vi "Kstar单相电界面.vi"() -> ()   [LabVIEW 2016, in "环境动力监测库.lvlib" / "UPS库.lvlib"]
panel:
  out "x+1":u32
  in  "解除告警":bool
  out "状态":T1
  out "通信":bool=TRUE
  out "串口":string
  in  "查看型号":bool
  out "关机倒计时":i32
  out "关闭中":bool
  out "UPS状态":T2
  in  "关机":bool
  in  "重开串口":bool
  # "输入电压"
  # "V"
  # "V"
  # "输入故障电压"
  # "输出电压"
  # "V"
  # "输出电流"
  # "A"
  # "输入频率"
  # "Hz"
  # "电池电压"
  # "V"
  # "UPS温度"
  # "℃"
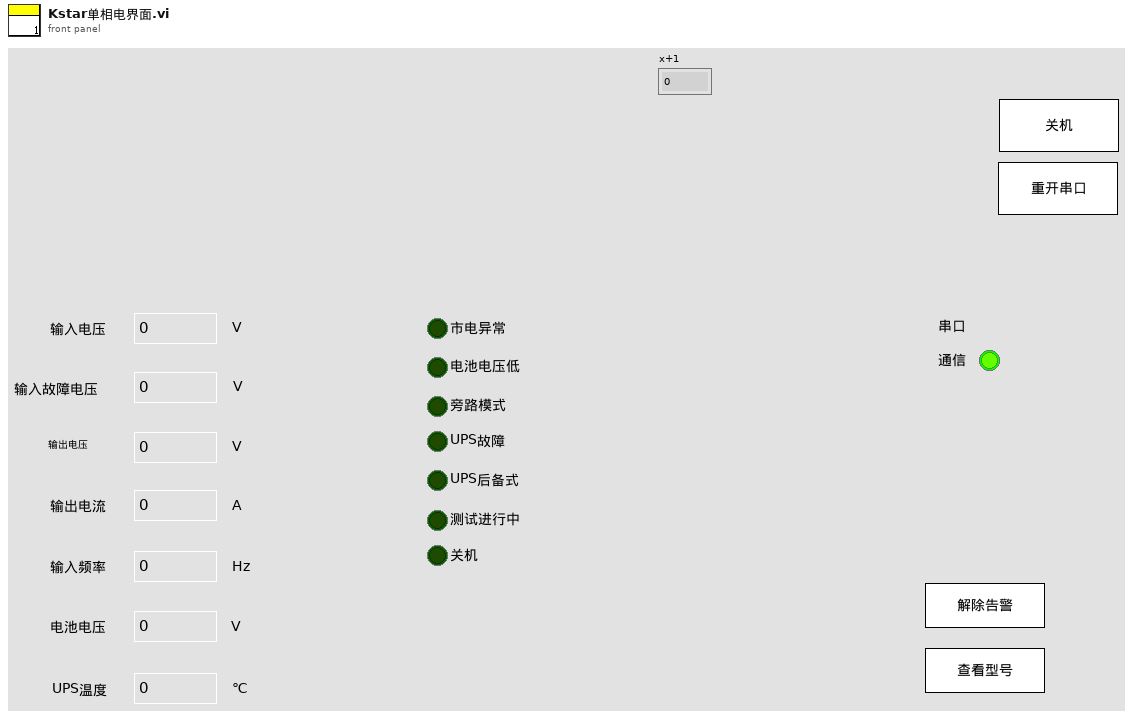
[diagram p1: front panel]
types:
  T1 = cluster{"I/P voltage":dbl, "I/P fault voltage":dbl, "O/P voltage":dbl, "O/P load %":dbl, "I/P frequency HZ":dbl, "Battery voltage":dbl, "Temperature":dbl}
  T2 = cluster{"市电异常":bool, "电池电压低":bool, "旁路模式":bool, "UPS故障":bool, "UPS后备式":bool, "测试进行中":bool, "关机":bool, "保留":bool}
  T3 = cluster{"枚举":enum16{"open", "read", "write", "close"}, "写入缓冲区":string}
  T4 = enum32{"Bad", "Idle", "Run top level", "Running"}
  T5 = cluster{"漏水监测输出":cluster{"漏水监测告警":bool, "告警内容":string}, "门禁监测输出":cluster{"门禁监测告警":bool, "告警内容":string}, "门禁监测输出2":cluster{"门禁监测告警":bool, "告警内容":string}, "温湿度监测输出":cluster{"温湿度监测告警":bool, "告警内容":string}, "烟雾监测输出":cluster{"烟雾监测告警":bool, "告警内容":string}, "空调监测输出":cluster{"空调监测告警":bool, "告警内容":string}, "自动重合闸输出":cluster{"自动重合闸告警":bool, "告警内容":string}, "红外入侵输出":cluster{"红外入侵告警":bool, "告警内容":string}, "振动输出":cluster{"振动告警":bool, "告警内容":string}, "UPS输出":cluster{"UPS告警":bool, "告警内容":string}, "蓄电池输出":cluster{"蓄电池告警":bool, "告警内容":string}, "蓄电池输出2":cluster{"蓄电池告警":bool, "告警内容":string}, "GPS输出":cluster{"定位告警":bool, "告警内容":string}, "北斗输出":cluster{"定位告警":bool, "告警内容":string}, "气象输出":cluster{"气象告警":bool, "告警内容":string}, "废液输出":cluster{"废液告警":bool, "告警内容":string}, "废液输出2":cluster{"废液告警":bool, "告警内容":string}, "灭火装置输出":cluster{"灭火装置告警":bool, "告警内容":string}}
  T6 = typedef "环境动力监测库.lvlib/UPS库.lvlib/UPS型号.ctl" = enum16{"山特UPSC1~3", "山特UPSC6~20", "华为UPS2000-G-(1-3KVA)", "Kstar"}
  T7 = cluster{"VISA resource name":refnum<visa-resource-name>, "Serial Config":cluster{"baud rate (9600)":u32, "stop bits (10: 1 bit)":u16, "parity (0:none)":enum16{"None", "Odd", "Even", "Mark", "Space"}, "data bits (8)":u16, "timeout (10sec)":u32}, "型号选择":T6, "HW-UPS-2000 MB session":refnum<class "MB_Master.lvclass">, "连接方式":enum16{"串口", "TCP"}, "IP":string, "Port":string, "低电量报警阈值":u16, "功能启用":bool}
  T8 = cluster{"I/P voltage":dbl, "I/P fault voltage":dbl, "O/P voltage":dbl, "O/P load %":dbl, "I/P frequency HZ":dbl, "Battery voltage":dbl, "Temperature":dbl, "U":string}
  T9 = cluster{"市电":cluster{"状态":bool, "电压:":u16, "电流：":dbl, "详情  ":bool}, "UPS":cluster{"状态":bool, "输入电压:":sgl, "输出电压:":sgl, "电池电量:":u8, "电量":u16, "详情  ":bool}, "蓄电池12V":cluster{"状态":bool, "电压:":sgl, "电流:":sgl, "电池电量:":u8, "电量":u16, "详情  ":bool, "充电":bool, "负载":bool}, "蓄电池24V":cluster{"状态":bool, "电压:":sgl, "电流:":sgl, "电池电量:":u8, "电量":u16, "详情  ":bool, "充电":bool, "负载":bool}}
  T10 = cluster{"[0]":bool, "[1]":bool, "[2]":bool, "[3]":bool, "[4]":bool, "[5]":bool, "[6]":bool, "[7]":bool}
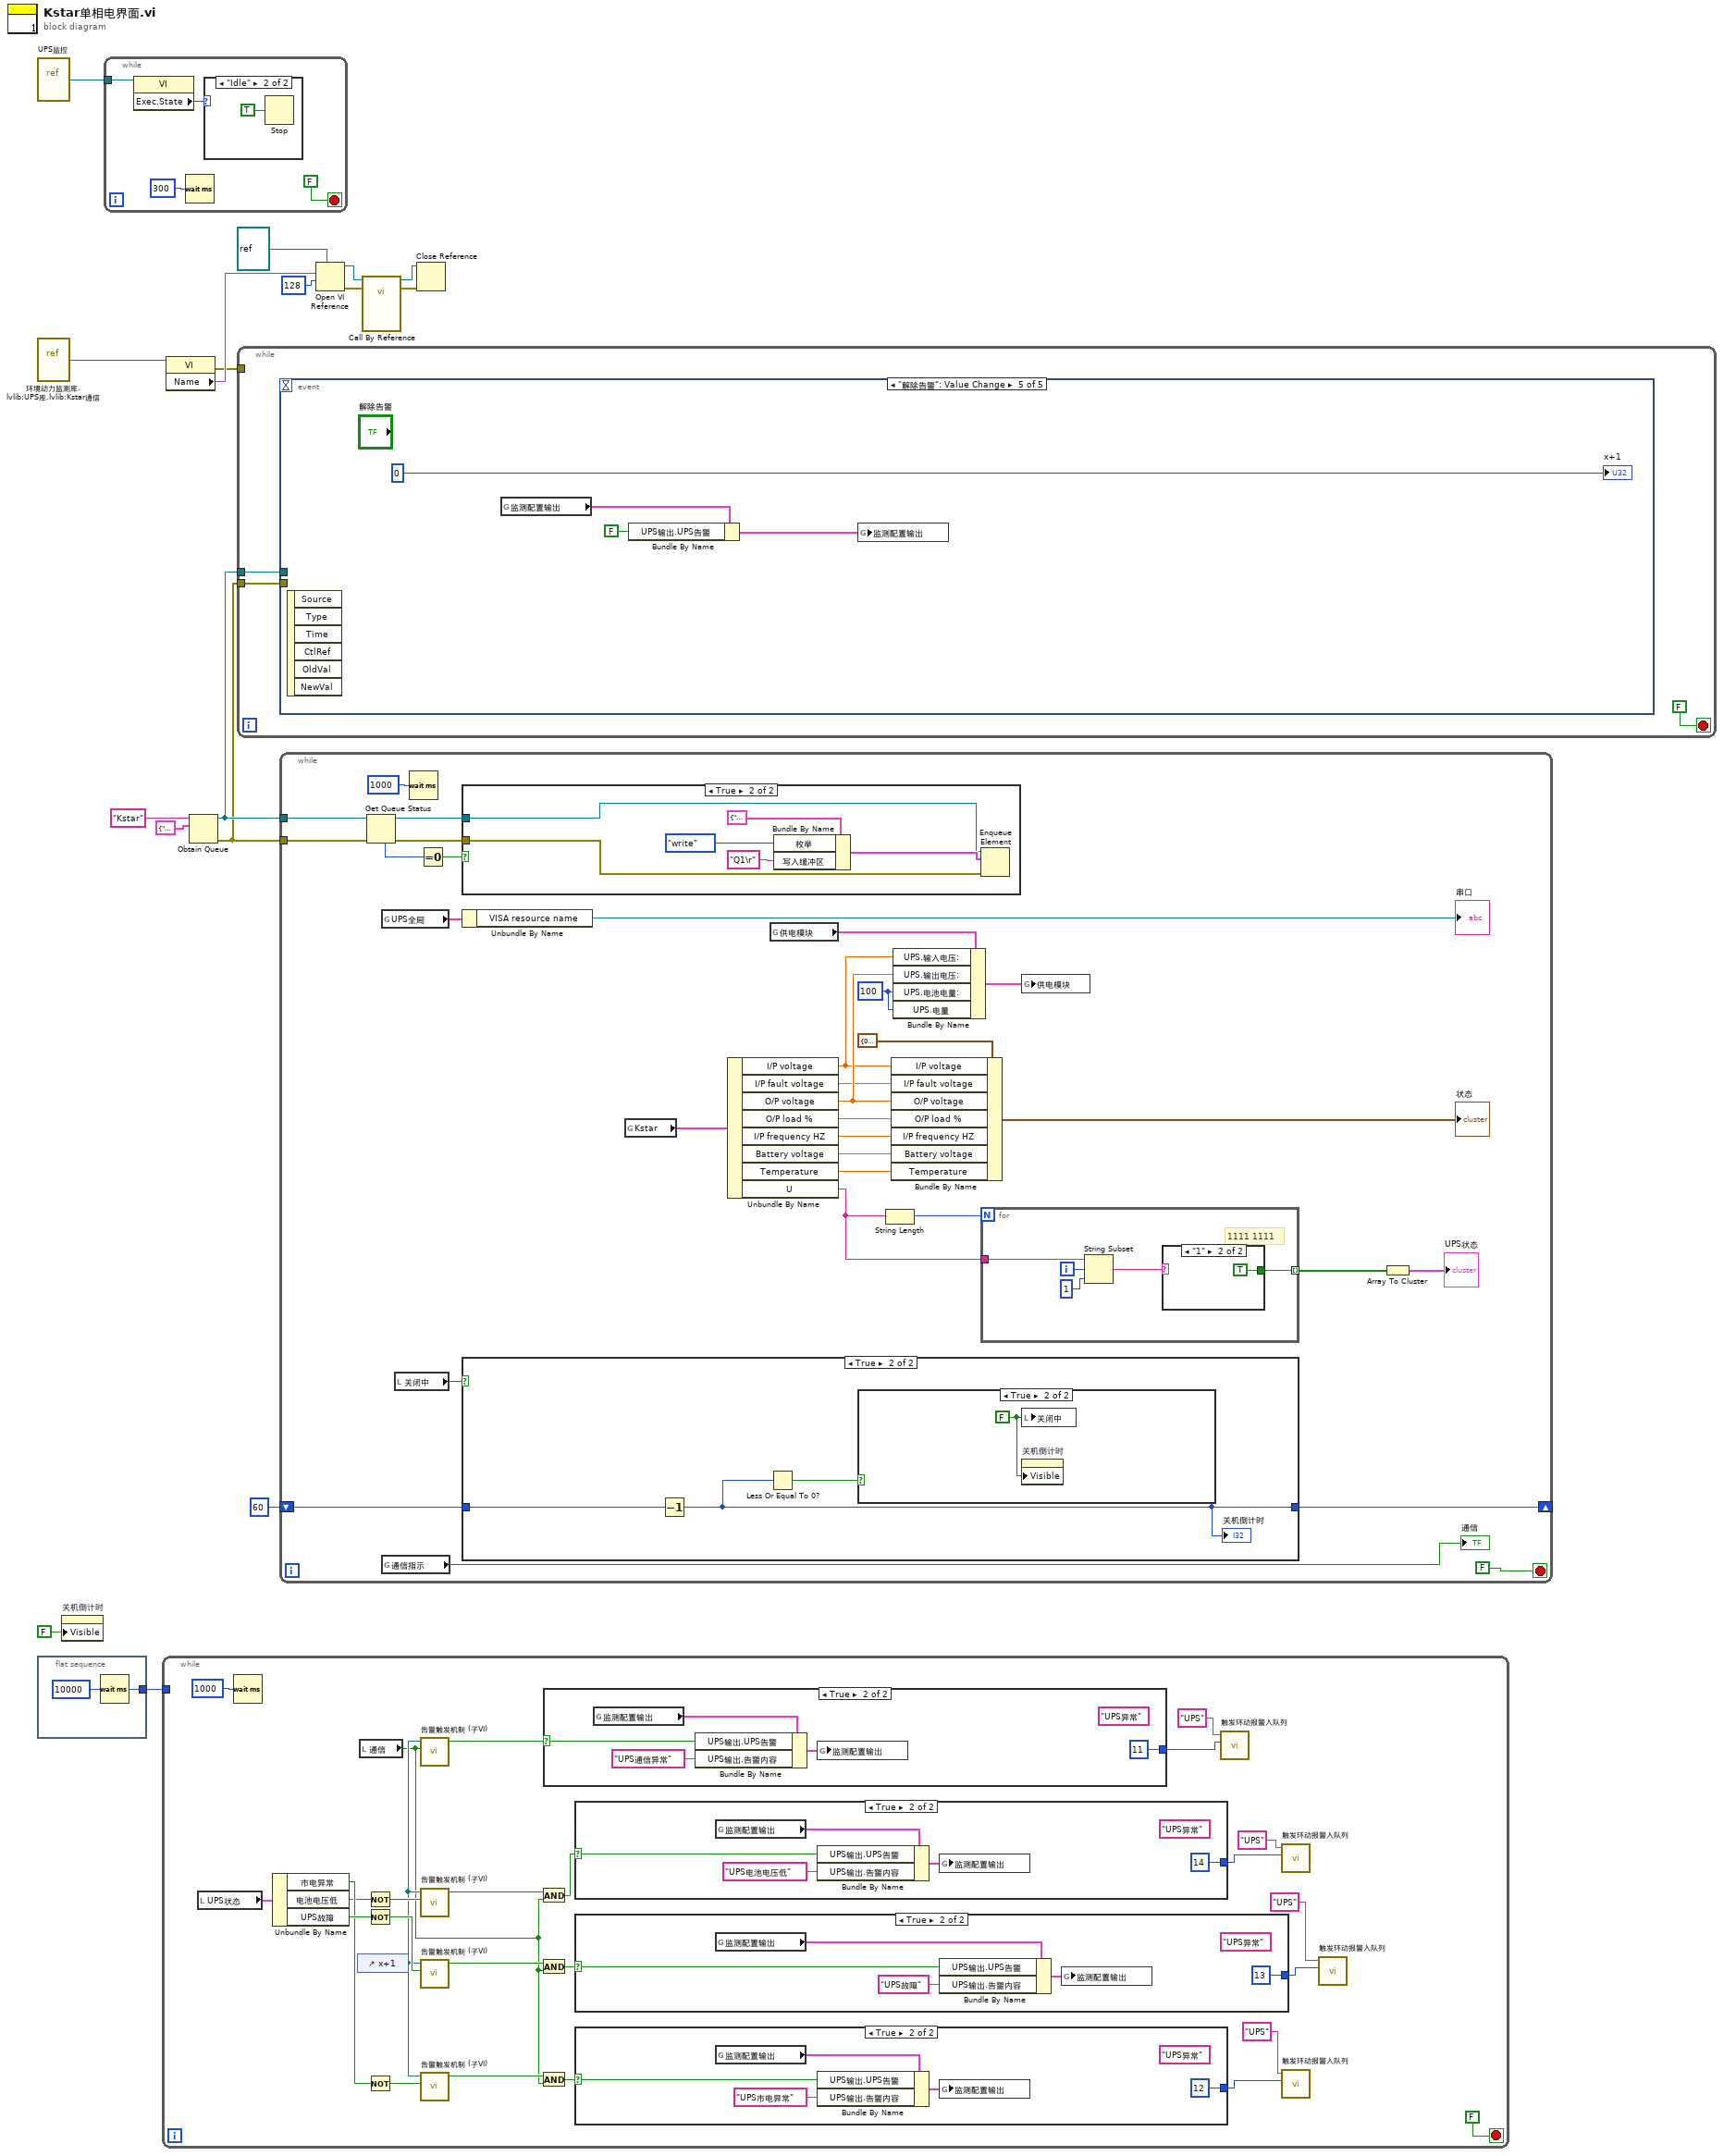
[diagram p0: block diagram]
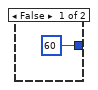
[diagram p8: hidden frame]
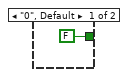
[diagram p10: hidden frame]
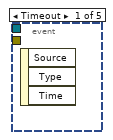
[diagram p11: hidden frame]
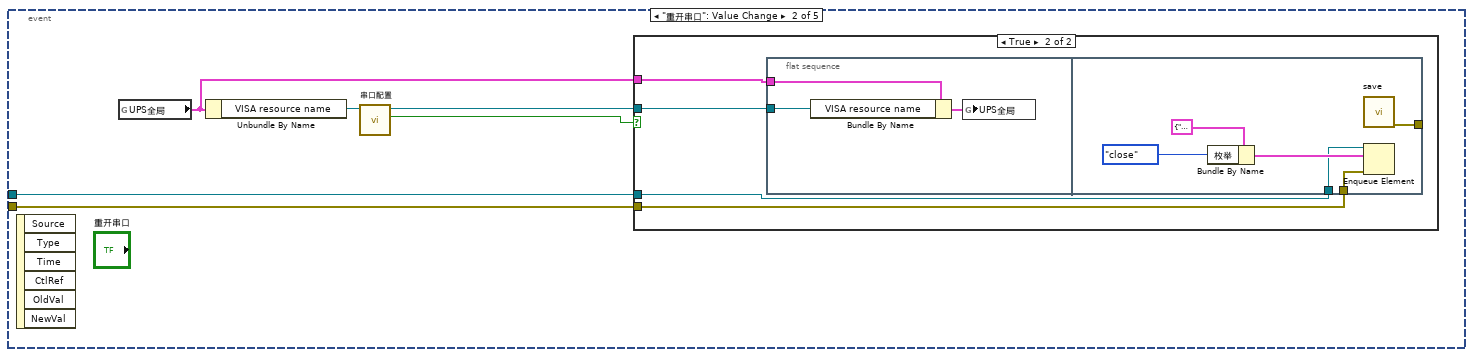
[diagram p12: hidden frame]
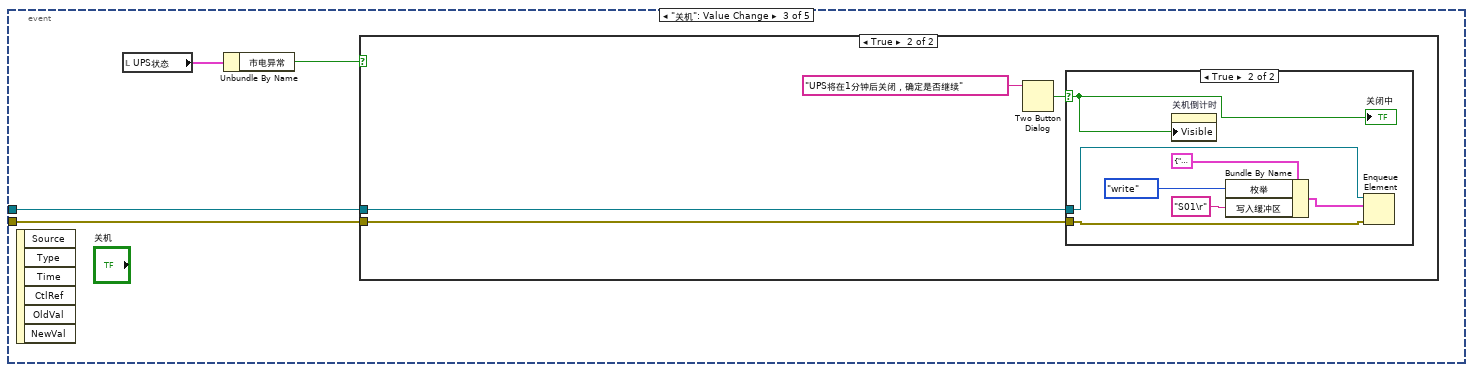
[diagram p14: hidden frame]
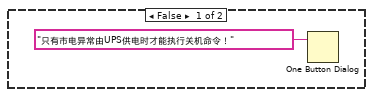
[diagram p15: hidden frame]
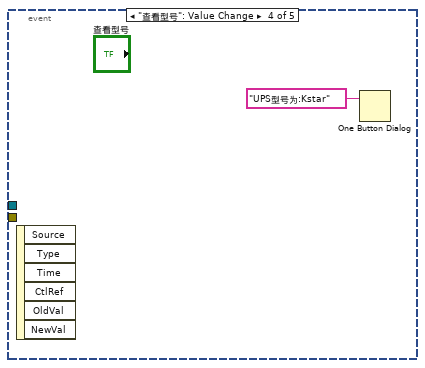
[diagram p17: hidden frame]
diagram:
  n1 = vi-ref "UPS监控.vi"() -> (w2:refnum<vi>)
  n2 = vi-ref "环境动力监测库.lvlib:UPS库.lvlib:Kstar通信.vi"() -> (w10:refnum<vi>)
  n3 = flat-sequence {
    tunnel: [w18] -> w1
    frame #0 {
      n4 = Wait (ms)(milliseconds to wait=u32 10000 ("等待时间（毫秒）")) -> (millisecond timer value=w18:u32)
    }
  }
  n5 = property on="关机倒计时" class="DigNum (strict)"("Visible"=FALSE ("可见")) -> ()  [unwired: 2 in, 2 out]
  n6 = while {
    tunnel: w2 -> [w23]
    stop <- FALSE stop-if-true
    n7 = property class="VI"(reference=w23) -> ("Exec.State"=w22:T4)  [unwired: 1 in, 2 out]
    n8 = Wait (ms)(milliseconds to wait=u32 300 ("等待时间（毫秒）")) -> ()  [unwired: 1 out]
    n9 = case shown="\"Idle\"" w22 {
      frame "Bad", Default {
      }
      frame "Idle" {
        n10 = Stop(stop? (T)=TRUE ("停止？(T)")) -> ()
      }
    }
  }
  n11 = while {
    tunnel: w1 -> [_]
    stop <- FALSE stop-if-true
    n12 = local read "UPS状态"() -> (w48:T2)
    n13 = Wait (ms)(milliseconds to wait=u32 1000 ("等待时间（毫秒）")) -> ()  [unwired: 1 out]
    n14 = Unbundle By Name(w48) -> ("市电异常"=w42:bool, "电池电压低"=w39:bool, "UPS故障"=w45:bool)
    n15 = control-ref of="x+1"() -> (w37:refnum<vi>)
    n16 = local read "通信"() -> (w33:bool)
    n17 = Not(x=w39) -> (.not. x?=w40:bool)
    n18 = Not(x=w45) -> (.not. x?=w46:bool)
    n19 = Not(x=w42) -> (.not. x?=w43:bool)
    n20 = call "告警触发机制 (子VI).vi"("状态输出真-正常"=w33, "Digital输入"=w37) -> ("触发告警"=w47:bool)  [unwired: 7 in, 2 out]
    n21 = call "告警触发机制 (子VI).vi"("状态输出真-正常"=w40, "Digital输入"=w37) -> ("触发告警"=w38:bool)  [unwired: 7 in, 2 out]
    n22 = call "告警触发机制 (子VI).vi"("状态输出真-正常"=w46, "Digital输入"=w37) -> ("触发告警"=w44:bool)  [unwired: 7 in, 2 out]
    n23 = call "告警触发机制 (子VI).vi"("状态输出真-正常"=w43, "Digital输入"=w37) -> ("触发告警"=w41:bool)  [unwired: 7 in, 2 out]
    n24 = And(x=w38, y=w33) -> (x .and. y?=w35:bool)
    n25 = And(x=w44, y=w33) -> (x .and. y?=w34:bool)
    n26 = And(x=w41, y=w33) -> (x .and. y?=w36:bool)
    n27 = case shown="True" w47 {
      selector: w47 -> [_ w55]
      tunnel: [_ 11 ("code")] -> w32
      frame False {
      }
      frame True {
        (unwired) "UPS异常" ("设备")
        n28 = global read "内部交互全局变量.vi" "监测配置输出"() -> (w53:T5)
        n29 = Bundle By Name(cluster=w53, "UPS输出.UPS告警"=w55, "UPS输出.告警内容"="UPS通信异常" ("报警内容")) -> (w54:T5)
        n30 = global write "内部交互全局变量.vi" "监测配置输出"(w54) -> ()
      }
    }
    n31 = case shown="True" w35 {
      selector: w35 -> [_ w65]
      tunnel: [_ 14 ("code")] -> w29
      frame False {
      }
      frame True {
        (unwired) "UPS异常" ("设备")
        n32 = global read "内部交互全局变量.vi" "监测配置输出"() -> (w64:T5)
        n33 = Bundle By Name(cluster=w64, "UPS输出.UPS告警"=w65, "UPS输出.告警内容"="UPS电池电压低" ("报警内容")) -> (w63:T5)
        n34 = global write "内部交互全局变量.vi" "监测配置输出"(w63) -> ()
      }
    }
    n35 = case shown="True" w34 {
      selector: w34 -> [_ w60]
      tunnel: [_ 13 ("code")] -> w28
      frame False {
      }
      frame True {
        (unwired) "UPS异常" ("设备")
        n36 = global read "内部交互全局变量.vi" "监测配置输出"() -> (w59:T5)
        n37 = Bundle By Name(cluster=w59, "UPS输出.UPS告警"=w60, "UPS输出.告警内容"="UPS故障" ("报警内容")) -> (w58:T5)
        n38 = global write "内部交互全局变量.vi" "监测配置输出"(w58) -> ()
      }
    }
    n39 = case shown="True" w36 {
      selector: w36 -> [_ w70]
      tunnel: [_ 12 ("code")] -> w27
      frame False {
      }
      frame True {
        (unwired) "UPS异常" ("设备")
        n40 = global read "内部交互全局变量.vi" "监测配置输出"() -> (w69:T5)
        n41 = Bundle By Name(cluster=w69, "UPS输出.UPS告警"=w70, "UPS输出.告警内容"="UPS市电异常" ("报警内容")) -> (w68:T5)
        n42 = global write "内部交互全局变量.vi" "监测配置输出"(w68) -> ()
      }
    }
    n43 = call "触发环动报警入队列.vi"("code"=w32, "元器件"="UPS" ("设备")) -> ()  [unwired: 10 in]
    n44 = call "触发环动报警入队列.vi"("code"=w29, "元器件"="UPS" ("设备")) -> ()  [unwired: 10 in]
    n45 = call "触发环动报警入队列.vi"("code"=w27, "元器件"="UPS" ("设备")) -> ()  [unwired: 10 in]
    n46 = call "触发环动报警入队列.vi"("code"=w28, "元器件"="UPS" ("设备")) -> ()  [unwired: 10 in]
  }
  n47 = property class="VI"(reference=w10) -> (error out=w4:errorcluster, "Name"=w11:string)  [unwired: 1 in, 1 out]
  n48 = Obtain Queue(name (unnamed)="Kstar" ("名称（未命名）"), element data type=T3 {"枚举"=enum."open", "写入缓冲区"=""}) -> (queue out=w7:refnum<queue>, error out=w6:errorcluster)  [unwired: 3 in, 1 out]
  n49 = while {
    tunnel: w6 -> [w72]
    tunnel: w7 -> [w71]
    tunnel: w4 -> [_]
    stop <- FALSE stop-if-true
    n50 = event shown="[4] \"解除告警\": Value Change" {
      selector: _ -> [_ _ _ _ _]
      dyn-events: _ -> [_ _ _ _ _]
      timeout: _ -> [_ _ _ _ _]
      tunnel: w72 -> [_ w76 w95 _ _]
      tunnel: w71 -> [_ w77 w96 _ _]
      event Timeout {
        n51 = event-data() -> ()  [unwired: 1 in, 3 out]
      }
      event "重开串口": Value Change {
        n52 = event-data() -> ()  [unwired: 1 in, 6 out]
        n53 = global read "断电保存全局变量.vi" "UPS全局"() -> (w74:T7)
        n54 = Unbundle By Name(w74) -> ("VISA resource name"=w75:refnum<visa-resource-name>)
        n55 = call "串口配置.vi"("请选择串口:"=w75) -> ("确认 2"=w79:bool, "请选择串口: 2"=w78:refnum<visa-resource-name>)  [unwired: 9 in]
        n56 = case shown="True" w79 {
          tunnel: w78 -> [_ w83]
          tunnel: w77 -> [_ w82]
          tunnel: w76 -> [_ w81]
          tunnel: w74 -> [_ w80]
          frame False {
          }
          frame True {
            n57 = flat-sequence {
              tunnel: w83 -> [w84]
              tunnel: w80 -> [w86]
              tunnel: w82 -> [w89]
              tunnel: w81 -> [w88]
              tunnel: [w87] -> _
              frame #0 {
                n58 = Bundle By Name(cluster=w86, "VISA resource name"=w84) -> (w85:T7)
                n59 = global write "断电保存全局变量.vi" "UPS全局"(w85) -> ()
              }
              frame #1 {
                n60 = Bundle By Name(cluster=T3 {"枚举"=enum."open", "写入缓冲区"=""}, "枚举"=enum16{"open", "read", "write", "close"}."close") -> (w92:T3)
                n61 = call "save.vi"() -> ("error out"=w87:errorcluster)  [unwired: 11 in]
                n62 = Enqueue Element(queue=w89, element=w92, error in (no error)=w88) -> ()  [unwired: 1 in, 3 out]
              }
            }
          }
        }
      }
      event "关机": Value Change {
        n63 = event-data() -> ()  [unwired: 1 in, 6 out]
        n64 = local read "UPS状态"() -> (w94:T2)
        n65 = Unbundle By Name(w94) -> ("市电异常"=w93:bool)
        n66 = case shown="True" w93 {
          tunnel: w96 -> [_ w101]
          tunnel: w95 -> [_ w100]
          frame False {
            n67 = One Button Dialog(message="只有市电异常由UPS供电时才能执行关机命令！" ("消息")) -> ()  [unwired: 1 in, 1 out]
          }
          frame True {
            n68 = Two Button Dialog(message="UPS将在1分钟后关闭，确定是否继续" ("消息")) -> (T button?=w98:bool)  [unwired: 2 in]
            n69 = case shown="True" w98 {
              selector: w98 -> [_ w102]
              tunnel: w101 -> [_ w105]
              tunnel: w100 -> [_ w104]
              frame False {
              }
              frame True {
                n70 = property on="关机倒计时" class="DigNum (strict)"("Visible"=w102) -> ()  [unwired: 2 in, 2 out]
                n71 = Bundle By Name(cluster=T3 {"枚举"=enum."open", "写入缓冲区"=""}, "枚举"=enum16{"open", "read", "write", "close"}."write", "写入缓冲区"="S01\r") -> (w106:T3)
                n72 = Enqueue Element(queue=w105, element=w106, error in (no error)=w104) -> ()  [unwired: 1 in, 3 out]
                "关闭中" <- w102
              }
            }
          }
        }
      }
      event "查看型号": Value Change {
        n73 = event-data() -> ()  [unwired: 1 in, 6 out]
        n74 = One Button Dialog(message="UPS型号为:Kstar" ("消息")) -> ()  [unwired: 1 in, 1 out]
      }
      event "解除告警": Value Change {
        n75 = event-data() -> ()  [unwired: 1 in, 6 out]
        n76 = global read "内部交互全局变量.vi" "监测配置输出"() -> (w111:T5)
        n77 = Bundle By Name(cluster=w111, "UPS输出.UPS告警"=FALSE) -> (w110:T5)
        n78 = global write "内部交互全局变量.vi" "监测配置输出"(w110) -> ()
        "x+1" <- u32 0 ("x+1")
      }
    }
  }
  n79 = while {
    tunnel: w7 -> [w134]
    tunnel: w6 -> [w133]
    shift-right: [w136] -> _
    shift-left: 60 -> [w137]
    stop <- FALSE stop-if-true
    w127 = u8 100 ("UPS.电池电量:")
    n80 = Get Queue Status(queue=w134, error in (no error)=w133) -> (queue out=w132:refnum<queue>, error out=w131:errorcluster, # elements in queue=w135:i32)  [unwired: 1 in, 5 out]
    n81 = global read "断电保存全局变量.vi" "UPS全局"() -> (w115:T7)
    n82 = global read "UPS内部交互全局.vi" "通信指示"() -> (→"通信":bool)
    n83 = local read "关闭中"() -> (w138:bool)
    n84 = Wait (ms)(milliseconds to wait=u32 1000 ("等待时间（毫秒）")) -> ()  [unwired: 1 out]
    n85 = Equal To 0?(x=w135) -> (x = 0?=w130:bool)
    n86 = case shown="True" w130 {
      tunnel: w132 -> [_ w146]
      tunnel: w131 -> [_ w145]
      frame False {
      }
      frame True {
        n87 = Bundle By Name(cluster=T3 {"枚举"=enum."open", "写入缓冲区"=""}, "枚举"=enum16{"open", "read", "write", "close"}."write", "写入缓冲区"="Q1\r") -> (w149:T3)
        n88 = Enqueue Element(queue=w146, element=w149, error in (no error)=w145) -> ()  [unwired: 1 in, 3 out]
      }
    }
    n89 = Unbundle By Name(w115) -> ("VISA resource name"=→"串口":refnum<visa-resource-name>)
    n90 = case shown="True" w138 {
      tunnel: w137 -> [_ w154]
      tunnel: [60 w153] -> w136
      frame False {
      }
      frame True {
        n91 = Decrement(x=w154) -> (x-1=w153:i32)
        "关机倒计时" <- w153
        n92 = Less Or Equal To 0?(x=w153) -> (x <= 0?=w152:bool)
        n93 = case shown="True" w152 {
          frame False {
          }
          frame True {
            w155 = FALSE ("关闭中")
            n94 = local write "关闭中"(w155) -> ()
            n95 = property on="关机倒计时" class="DigNum (strict)"("Visible"=w155) -> ()  [unwired: 2 in, 2 out]
          }
        }
      }
    }
    n96 = global read "UPS内部交互全局.vi" "Kstar"() -> (w142:T8)
    n97 = Unbundle By Name(w142) -> ("I/P voltage"=w117:dbl, "I/P fault voltage"=w116:dbl, "O/P voltage"=w118:dbl, "O/P load %"=w119:dbl, "I/P frequency HZ"=w120:dbl, "Battery voltage"=w121:dbl, "Temperature"=w122:dbl, "U"=w139:string)
    n98 = global read "内部交互全局变量.vi" "供电模块"() -> (w129:T9)
    n99 = String Length(string=w139) -> (length=w140:i32)
    n100 = Bundle By Name(cluster=T1 {"I/P voltage"=0.0, "I/P fault voltage"=0.0, "O/P voltage"=0.0, "O/P load %"=0.0, "I/P frequency HZ"=0.0, "Battery voltage"=0.0, "Temperature"=0.0} ("状态"), "I/P voltage"=w117, "I/P fault voltage"=w116, "O/P voltage"=w118, "O/P load %"=w119, "I/P frequency HZ"=w120, "Battery voltage"=w121, "Temperature"=w122) -> (→"状态":T1)
    n101 = Bundle By Name(cluster=w129, "UPS.输入电压:"=w117, "UPS.输出电压:"=w118, "UPS.电池电量:"=w127, "UPS.电量"=w127) -> (w128:T9)
    n102 = for {
      N: w140 -> [_]
      tunnel: w139 -> [w160]
      tunnel: [w156] -> w126 mode=indexing
      i -> [w158]
      # "1111 1111"
      n103 = String Subset(string=w160, offset (0)=w158, length (rest)=1 ("长度（剩余）")) -> (substring=w157:string)
      n104 = case shown="\"1\"" w157 {
        tunnel: [FALSE TRUE] -> w156
        frame "0", Default {
        }
        frame "1" {
        }
      }
    }
    n105 = global write "内部交互全局变量.vi" "供电模块"(w128) -> ()
    n106 = Array To Cluster(array=w126) -> (cluster=→"UPS状态":T10)
  }
  n107 = Open VI Reference(type specifier VI Refnum (for type only)=refnum<vi> refnum, vi path=w11, options=128 ("选项")) -> (vi reference=w13:refnum<vi>, error out=w15:errorcluster)  [unwired: 3 in]
  n108 = call-by-ref "?"(reference=w13, error in=w15) -> (reference out=w17:refnum<vi>, error out=w16:errorcluster)  [unwired: 12 in]
  n109 = Close Reference(reference=w17, error in (no error)=w16) -> ()  [unwired: 1 out]
